vi "dllErrorCodeToLabVIEWError.vi"(8 "error in (no error)":errorcluster, 10 "error code in":u32, 11 "ActiveMQBroker in":refnum<class "ActiveMQBroker.lvclass">) -> (0 "error out":errorcluster, 3 "ActiveMQBroker out":refnum<class "ActiveMQBroker.lvclass">)   [LabVIEW 2012, in "ActiveMQBroker.lvclass"]
doc: "Convert error codes returned by dll to LabVIEW error datatype."
uses:
  <userlib>/Common/Communication/ActiveMQ/ActiveMQBroker/ActiveMQBroker.lvclass
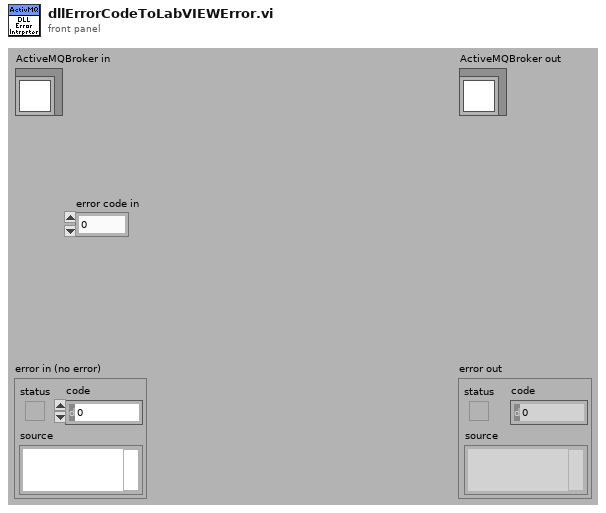
[diagram p1: front panel]
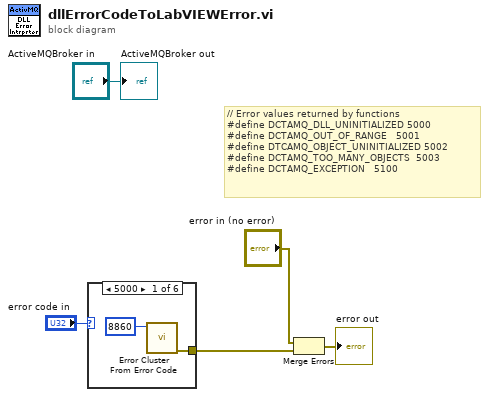
[diagram p0: block diagram]
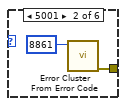
[diagram p2: hidden frame]
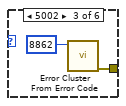
[diagram p3: hidden frame]
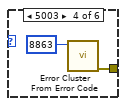
[diagram p4: hidden frame]
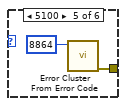
[diagram p5: hidden frame]
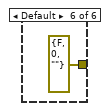
[diagram p6: hidden frame]
diagram:
  # "// Error values returned by functions\n#define DCTAMQ_DLL_UNINITIALIZED\t5000\n#define DCTAMQ_OUT_OF_RANGE\t\t\t5001\n#define DTCAMQ_OBJECT_UNINITIALIZED\t5002\n#define DCTAMQ_TOO_MANY_OBJECTS\t\t5003\n#define DCTAMQ_EXCEPTION\t\t\t5100"
  n1 = case shown="5000" "error code in" {
    tunnel: [w6 w8 w10 w12 w14 errorcluster {"status"=FALSE, "code"=0, "source"=""} ("error out")] -> w2
    frame 5000 {
      n2 = call <vilib>:"Error Cluster From Error Code.vi"("error code (0)"=8860) -> ("error out"=w6:errorcluster)  [unwired: 8 in]
    }
    frame 5001 {
      n3 = call <vilib>:"Error Cluster From Error Code.vi"("error code (0)"=8861) -> ("error out"=w8:errorcluster)  [unwired: 8 in]
    }
    frame 5002 {
      n4 = call <vilib>:"Error Cluster From Error Code.vi"("error code (0)"=8862) -> ("error out"=w10:errorcluster)  [unwired: 8 in]
    }
    frame 5003 {
      n5 = call <vilib>:"Error Cluster From Error Code.vi"("error code (0)"=8863) -> ("error out"=w12:errorcluster)  [unwired: 8 in]
    }
    frame 5100 {
      n6 = call <vilib>:"Error Cluster From Error Code.vi"("error code (0)"=8864) -> ("error out"=w14:errorcluster)  [unwired: 8 in]
    }
    frame Default {
    }
  }
  n7 = Merge Errors("error in (no error)", w2) -> (→"error out":errorcluster)
  "ActiveMQBroker out" <- "ActiveMQBroker in"
